vi "force_close.vi"   [LabVIEW 2015]
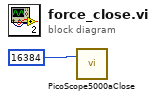
[diagram p0: block diagram]
diagram:
  n1 = call "PicoScope5000aClose.vi"("handle"=i16 16384) -> ()  [unwired: 2 in, 1 out]
